vi "initialise.vi"(8 "error in (no error)":errorcluster, 11 "GenericPlugin in":refnum<class "FPGAWrapperMH120124FrameScan_PXI7813R.lvclass">) -> (0 "error out":errorcluster, 3 "GenericPlugin out":refnum<class "FPGAWrapperMH120124FrameScan_PXI7813R.lvclass">)   [LabVIEW 2010, in "FPGAWrapperMH120124FrameScan_PXI7813R.lvclass"]
doc: "The dynamic dispatch-version of this VI initalises the plug-in object by allocating and initalising any dynamic resources need."
uses:
  FPGAWrapperMH120124FrameScan_PXI7813R.lvclass
  GenericFPGAWrapper/GenericFPGAWrapper/GenericFPGAWrapper.lvclass
  grabber/command_enum.ctl
  FPGAWrapperMH120124FrameScan_PXI7813R.lvclass/FPGAWrapperMH120124FrameScan_PXI7813R.ctl
  class_data.vi
  common/classes/ErrorController/ErrorController/class_data.vi
  common/classes/ErrorController/ErrorController/ErrorController.lvclass
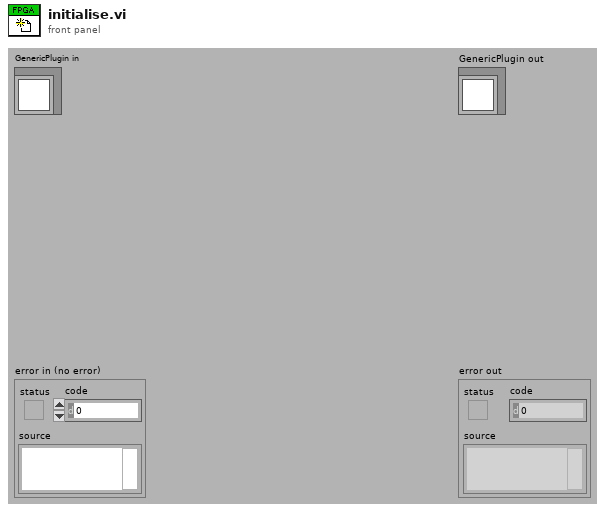
[diagram p1: front panel]
types:
  T1 = typedef "command_enum.ctl" = enum8{"NULL", "update", "start", "stop", "reset", "shut-down"}
  T2 = typedef "configuration_cluster_framescan.ctl" = cluster{"DDS board initialization parameters":T3, "OSK select":bool, "inverse?":string, "AOD equilibration time":dbl, "AOD amplitude":u16, "AOD center frequ. (Hz)":dbl, "AOD Bandwidth":dbl}
  T3 = typedef "DDS_board_init_cluster.ctl" = cluster{"Bypass PLL":bool, "PLL Range":bool, "Update Clock":bool, "Triangle ":bool, "SDO Active":bool, "LSB First":bool, "OSK Int":bool, "Output Shaped Keying Enable":bool, "Bypass Sinc":bool, "Digital Part":bool, "OutPut DAC":bool, "Control DAC":bool, "Comparator":bool, "Modus":u8, "Multiplier Value":u8}
  T4 = typedef "settings_cluster_framescan.ctl" = cluster{"number of pixels":i32, "iterations per pixel":i32, "maximum bit-depth":i8, "AOD center freq. (Hz)":dbl, "AOD bandwidth freq. (Hz)":dbl, "AOD amplitude":dbl, "pixel dwell time":dbl, "AOD equilibration time":dbl, "x resolution":i32, "y resolution":i32, "z angle (rotation angle, phi)":dbl, "x angle (tilting angle, phi)":dbl, "zoom":dbl, "pixel values cluster":T5, "offset (Hz)":dbl[], "DDS board initialization parameters":T3}
  T5 = typedef "channels_cluster.ctl" = cluster{"channel 0":u32, "channel 1":u32, "channel 2":u32, "channel 3":u32}
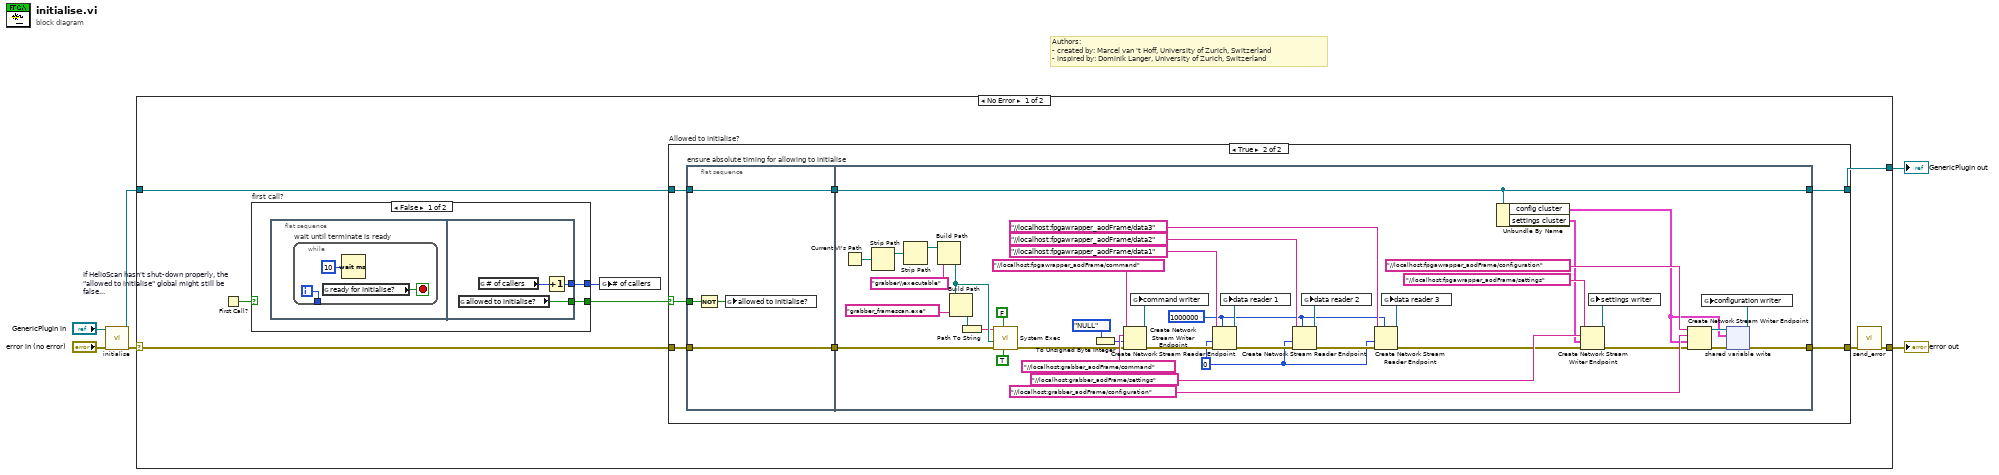
[diagram p0: block diagram]
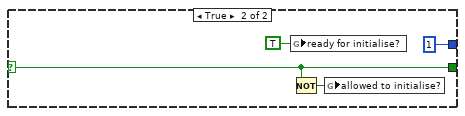
[diagram p2: hidden frame]
diagram:
  # "Authors: \n- created by: Marcel van 't Hoff, University of Zurich, Switzerland\n- inspired by: Dominik Langer, University of Zurich, Switzerland"
  n1 = call-parent "initialise.vi"("error in (no error)"="error in (no error)", "GenericPlugin in"="GenericPlugin in") -> ("error out"=w4:errorcluster, "GenericPlugin out"=w3:refnum<class "FPGAWrapperMH120124FrameScan_PXI7813R.lvclass">)  [unwired: 8 in]
  n2 = case shown="No Error" w4 {
    selector: w4 -> [w7 w83]
    tunnel: w3 -> [w11 w82]
    tunnel: [w14 w82] -> w2
    tunnel: [w13 w83] -> w1
    frame No Error {
      n3 = First Call? "If HelioScan hasn't shut-down properly, the \"allowed to initialise\" global might still be false..."() -> (First Call?: T/F=w10:bool)
      n4 = case "first call?" shown="False" w10 {
        selector: w10 -> [_ w25]
        tunnel: [w15 w25] -> w8
        tunnel: [w16 1 ("# of callers")] -> w9
        frame False {
          n5 = flat-sequence {
            tunnel: [w21] -> w16
            tunnel: [w20] -> w15
            frame #0 {
              n6 = while "wait until terminate is ready" {
                tunnel: [w17] -> _
                i -> [w17]
                stop <- w19 stop-if-true
                n7 = global read "class_data.vi" "ready for initialise?"() -> (w19:bool)
                n8 = Wait (ms)(milliseconds to wait=u32 10) -> ()  [unwired: 1 out]
              }
            }
            frame #1 {
              n9 = global read "class_data.vi" "allowed to initialise?"() -> (w20:bool)
              n10 = global read "class_data.vi" "# of callers"() -> (w22:i32)
              n11 = Increment(x=w22) -> (x+1=w21:i32)
            }
          }
        }
        frame True {
          n12 = global write "class_data.vi" "ready for initialise?"(TRUE ("ready for initialise?")) -> ()
          n13 = Not(x=w25) -> (.not. x?=w24:bool)
          n14 = global write "class_data.vi" "allowed to initialise?"(w24) -> ()
        }
      }
      n15 = global write "class_data.vi" "# of callers"(w9) -> ()
      n16 = case "Allowed to initialise?" shown="True" w8 {
        selector: w8 -> [_ w29]
        tunnel: [w27 w30] -> w14
        tunnel: w11 -> [w27 w31]
        tunnel: [w28 w34] -> w12
        tunnel: w7 -> [w28 w35]
        frame False {
        }
        frame True {
          n17 = flat-sequence "ensure absolute timing for allowing to initialise" {
            tunnel: w31 -> [w38]
            tunnel: w35 -> [w39]
            tunnel: [w39] -> w33
            tunnel: [w38] -> w32
            tunnel: w29 -> [w37]
            tunnel: [w54] -> w34
            tunnel: w33 -> [w81]
            tunnel: w32 -> [w40]
            tunnel: [w40] -> w30
            frame #0 {
              n18 = Not(x=w37) -> (.not. x?=w36:bool)
              n19 = global write "class_data.vi" "allowed to initialise?"(w36) -> ()
            }
            frame #1 {
              w56 = 1000000 ("reader buffer size")
              w63 = u32 0
              n20 = Current VI's Path() -> (path=w45:path)
              n21 = Strip Path(path=w45) -> (stripped path=w42:path)  [unwired: 1 out]
              n22 = Strip Path(path=w42) -> (stripped path=w41:path)  [unwired: 1 out]
              n23 = Build Path(base path=w41, name or relative path="grabber\\executable") -> (appended path=w48:path)
              n24 = Build Path(base path=w48, name or relative path="grabber_framescan.exe" ("command line")) -> (appended path=w47:path)
              n25 = Path To String(path=w47) -> (string=w46:string)
              n26 = call <vilib>:"System Exec.vi"("run minimized? (F)"=TRUE, "wait until completion? (T)"=FALSE, "error in (no error)"=w81, "working directory"=w48, "command line"=w46) -> ("error out"=w69:errorcluster)  [unwired: 3 in, 3 out]
              n27 = To Unsigned Byte Integer(number=command_enum."NULL" ("command")) -> (unsigned 8bit integer=w58:u8)
              n28 = Create Network Stream Writer Endpoint(8:w69, 9:w58, 10:"//localhost:grabber_aodFrame/command" ("writer name"), 11:"//localhost:fpgawrapper_aodFrame/command" ("writer name")) -> (0:w72:errorcluster, 3:w57:refnum<k21>)  [unwired: 2 in]
              n29 = global write "class_data.vi" "command writer"(w57) -> ()
              n30 = Create Network Stream Reader Endpoint(7:w56, 8:w72, 9:w63, 11:"//localhost:fpgawrapper_aodFrame/data1" ("reader url")) -> (0:w66:errorcluster, 3:w60:refnum<k21>)  [unwired: 2 in]
              n31 = global write "class_data.vi" "data reader 1"(w60) -> ()
              n32 = Create Network Stream Reader Endpoint(7:w56, 8:w66, 9:w63, 11:"//localhost:fpgawrapper_aodFrame/data2" ("reader url")) -> (0:w67:errorcluster, 3:w62:refnum<k21>)  [unwired: 2 in]
              n33 = global write "class_data.vi" "data reader 2"(w62) -> ()
              n34 = Create Network Stream Reader Endpoint(7:w56, 8:w67, 9:w63, 11:"//localhost:fpgawrapper_aodFrame/data3" ("reader url")) -> (0:w55:errorcluster, 3:w61:refnum<k21>)  [unwired: 2 in]
              n35 = global write "class_data.vi" "data reader 3"(w61) -> ()
              n36 = Unbundle By Name(w40) -> ("config cluster"=w52:T2, "settings cluster"=w68:T4)
              n37 = Create Network Stream Writer Endpoint(8:w55, 9:w68, 10:"//localhost:grabber_aodFrame/settings" ("writer name"), 11:"//localhost:fpgawrapper_aodFrame/settings" ("writer name")) -> (0:w76:errorcluster, 3:w53:refnum<k21>)  [unwired: 2 in]
              n38 = global write "class_data.vi" "settings writer"(w53) -> ()
              n39 = Create Network Stream Writer Endpoint(8:w76, 9:w52, 10:"//localhost:grabber_aodFrame/configuration" ("reader url"), 11:"//localhost:fpgawrapper_aodFrame/configuration" ("writer name")) -> (0:w75:errorcluster, 3:w74:refnum<k21>)  [unwired: 2 in]
              n40 = shared-variable-write(w74, w75, w52) -> (w51:refnum<k21>, w54:errorcluster)  [unwired: 1 in, 1 out]
              n41 = global write "class_data.vi" "configuration writer"(w51) -> ()
            }
          }
        }
      }
      n42 = call "send_error.vi"("error in (no error)"=w12) -> ("error out"=w13:errorcluster)  [unwired: 10 in]
    }
    frame Error {
    }
  }
  "error out" <- w1
  "GenericPlugin out" <- w2
